vi "Initialize CSV.vi"(8 "error in (no error)":errorcluster, 11 "Settings IN":T1={"State"=enum."Idle S3DK", "Settings"="", "Online"=FALSE, "S3DK"={"Signals"={"Phasor"=[], "Analog"=[], "Digital"=[]}}, "CSV"={"CSV Path"=path "", "Index"=0, "Parcel Length"=0, "EOF?"=FALSE}}) -> (0 "error out":errorcluster, 3 "Settings OUT":T1={"State"=enum."Idle S3DK", "Settings"="", "Online"=FALSE, "S3DK"={"Signals"={"Phasor"=[], "Analog"=[], "Digital"=[]}}, "CSV"={"CSV Path"=path "", "Index"=0, "Parcel Length"=0, "EOF?"=FALSE}})   [LabVIEW 2017, in "Acquisition.lvlib"]
doc: "Initialize the hardware references."
uses:
  Acquisition.lvlib
  Acquisition Settings.ctl
  Acquisition State.ctl
  <vilib>/Utility/file.llb/Read Delimited Spreadsheet (DBL).vi
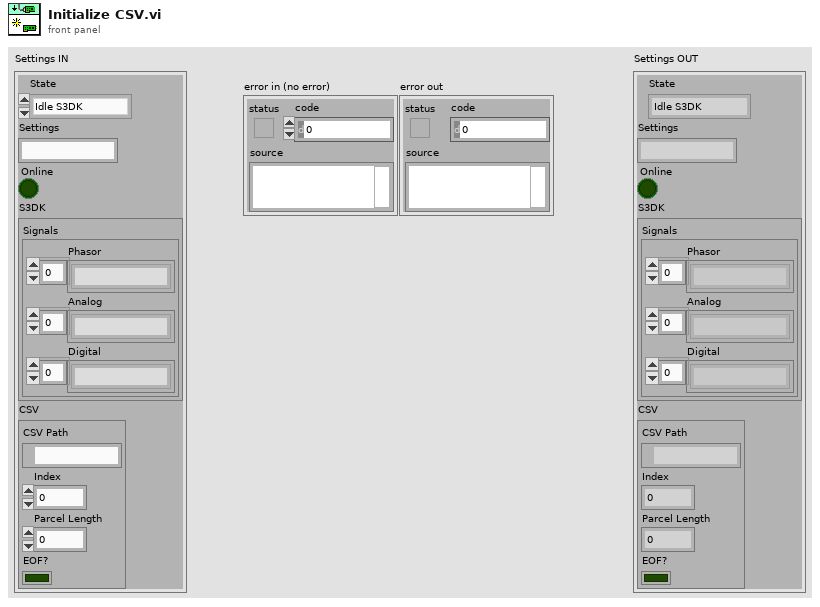
[diagram p1: front panel]
types:
  T1 = typedef "Acquisition.lvlib/Acquisition Settings.ctl" = cluster{"State":T2, "Settings":string, "Online":bool, "S3DK":cluster{"Signals":cluster{"Phasor":string[], "Analog":string[], "Digital":string[]}}, "CSV":cluster{"CSV Path":path, "Index":i32, "Parcel Length":i32, "EOF?":bool}}
  T2 = typedef "Acquisition.lvlib/Acquisition State.ctl" = enum16{"Idle", "Idle S3DK", "Acquiring S3DK", "Idle CSV", "Acquiring CSV"}
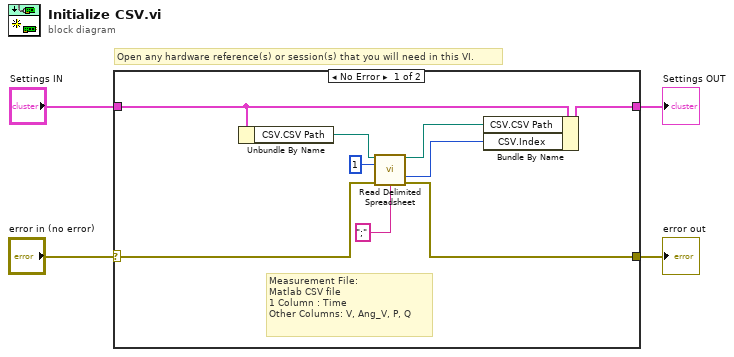
[diagram p0: block diagram]
diagram:
  # "Open any hardware reference(s) or session(s) that you will need in this VI."
  n1 = case shown="No Error" "error in (no error)" {
    selector: "error in (no error)" -> [w5 w14]
    tunnel: [w10 w14] -> w3
    tunnel: "Settings IN" -> [w7 w15]
    tunnel: [w13 w15] -> w1
    frame No Error {
      # "Measurement File:\nMatlab CSV file\n1 Column : Time \nOther Columns: V, Ang_V, P, Q"
      n2 = Unbundle By Name(w7) -> ("CSV.CSV Path"=w6:path)
      n3 = call-poly <vilib>:"Read Delimited Spreadsheet.vi"("file path (dialog if empty)"=w6, "number of rows (all:-1)"=1, "error in (no error)"=w5, "delimiter (\\t)"=";" ("delimiter (\\t)")) -> ("new file path (Not A Path if cancelled)"=w12:path, "mark after read (chars.)"=w8:i32, "error out"=w10:errorcluster)  [unwired: 6 in, 3 out]
      n4 = Bundle By Name(cluster=w7, "CSV.CSV Path"=w12, "CSV.Index"=w8) -> (w13:T1)
    }
    frame Error {
    }
  }
  "Settings OUT" <- w1
  "error out" <- w3
